vi "Actor Core.vi"(8 "error in":errorcluster, 11 "WS Test Client in":refnum<class "WS Test Client Subscriber.lvclass">) -> (0 "error out":errorcluster, 3 "Actor out":refnum<class "Actor.lvclass">)   [LabVIEW 2017, in "Echo Broadcast Test With Server Manager.lvlib" / "WS Test Client Subscriber.lvclass"]
doc: "(<B>Filename</B>: Actor Framework.lvlib:Actor.lvclass:Actor Core.vi)\n\nReceives messages to the actor, reacts to them, and initiates any error handling that may shut the actor down.\n\nDescendant classes may override this VI to append parallel tasks for the actor to complete while it handles messages. Overrides use the Call Parent Method node."
uses:
  WS Test Client Subscriber.lvclass
  C:/Program Files (x86)/National Instruments/LabVIEW 2017/vi.lib/ActorFramework/Actor/Actor.lvclass
  <vilib>/ActorFramework/Actor/Actor.lvclass
  <vilib>/ActorFramework/Message Enqueuer/Message Enqueuer.lvclass
  WebSocket Actor/WebSocket Client/WebSocket Client.lvclass
  C:/Projects/Shared Libraries/WebSocket Actor/WebSocket Actor/WebSocket Connection/WebSocket Connection.lvclass
  WS Test Client Subscriber Messages/Client Connection Handler Msg/Client Connection Handler Msg.lvclass
  C:/Projects/Shared Libraries/WebSocket Actor/WebSocket Actor/Abstract Messages/WebSocket Connection Handler Msg/WebSocket Connection Handler Msg.lvclass
  <vilib>/ActorFramework/Actor/Actor.lvclass/Actor.ctl
  <vilib>/ActorFramework/Message Enqueuer/Message Enqueuer.lvclass/Message Enqueuer.ctl
  WebSocket Actor/WebSocket Client/WebSocket Client.lvclass/WebSocket Client.ctl
  WebSocket Actor/WebSocket Connection/WebSocket Connection.lvclass/WebSocket Connection.ctl
  WS Test Client Subscriber.lvclass/WS Test Client Subscriber.ctl
  WebSocket Actor/WebSocket Client/properties/Write WS URI.vi
  WebSocket Actor/WebSocket Connection/properties/Write Timeout.vi
  WebSocket Actor/WebSocket Connection/properties/Write WebSocket Data Handler.vi
  <vilib>/ActorFramework/Message Enqueuer/Init from Existing Queue.vi
  <vilib>/ActorFramework/Message Enqueuer/Enqueue.vi
  <vilib>/ActorFramework/Stop Msg/Stop Msg.lvclass
  C:/Program Files (x86)/National Instruments/LabVIEW 2017/vi.lib/ActorFramework/Message/Message.lvclass
  <vilib>/ActorFramework/Message Priority Queue/Priority Enqueue.vi
  <vilib>/MGI/Monitored Actor/Monitored Actor/Monitored Actor/Monitored Actor.lvclass
  WebSocket Actor/WebSocket Connection Messages/Send to Peer Msg/Send to Peer Msg.lvclass
panel:
  in  "Send":bool
  in  "Data To Send":string
  in  "Exit":bool
  out "Echoed Data":string
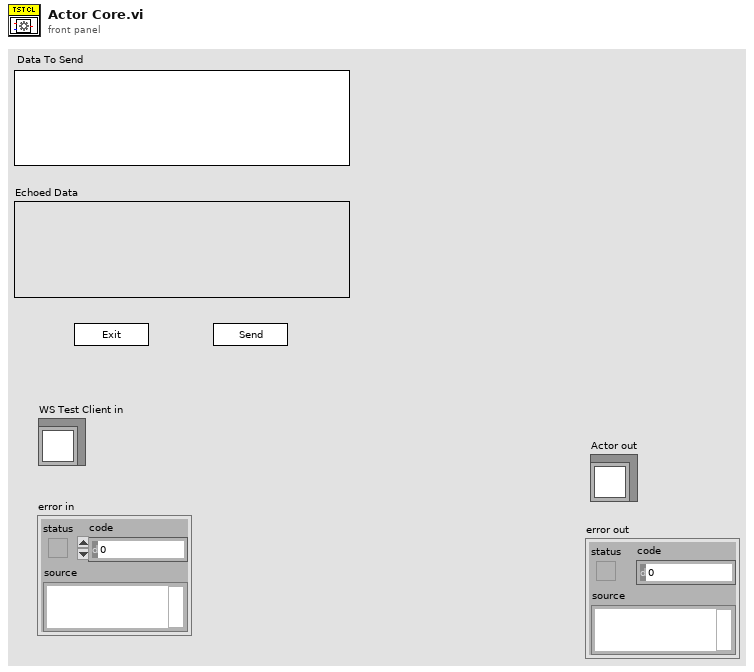
[diagram p1: front panel]
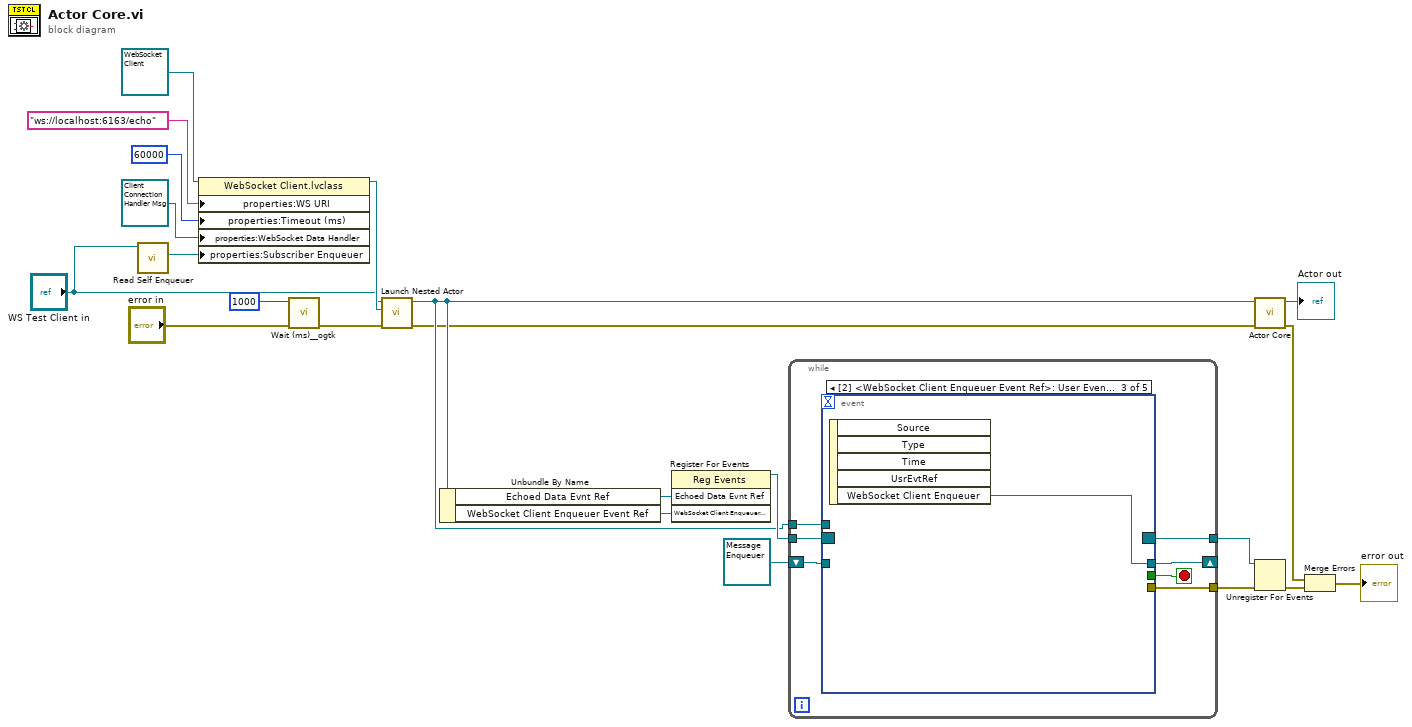
[diagram p0: block diagram]
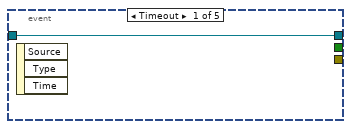
[diagram p2: hidden frame]
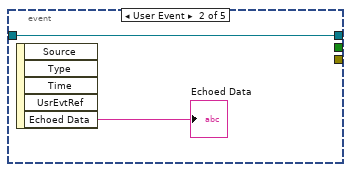
[diagram p3: hidden frame]
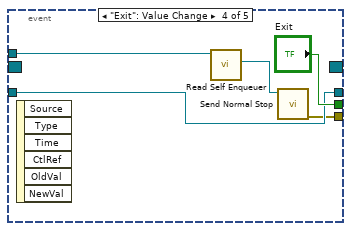
[diagram p4: hidden frame]
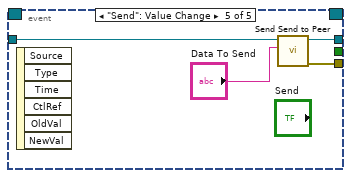
[diagram p5: hidden frame]
diagram:
  n1 = call <vilib>:"Read Self Enqueuer.vi"("Actor"="WS Test Client in") -> ("Self Enqueuer"=w5:refnum<class "Message Enqueuer.lvclass">)  [unwired: 10 in]
  n2 = property class="WebSocket Client.lvclass"(reference=refnum<class "WebSocket Client.lvclass"> refnum ("WebSocket Actors.lvlib:WebSocket Client.lvclass"), "properties:WS URI"="ws://localhost:6163/echo" ("Address"), "properties:Timeout (ms)"=60000 ("Timeout (60000 ms)"), "properties:WebSocket Data Handler"=refnum<class "Client Connection Handler Msg.lvclass"> refnum ("WS Full LabVIEW Test.lvlib:Client Connection Handler Msg.lvclass"), "properties:Subscriber Enqueuer"=w5) -> (reference out=w10:refnum<class "WebSocket Client.lvclass">)  [unwired: 1 in, 1 out]
  n3 = call <userlib>:"Wait (ms)__ogtk.vi"("error in (no error)"="error in", "milliseconds to wait"=u32 1000) -> ("error out"=w7:errorcluster)  [unwired: 8 in, 1 out]
  n4 = call <vilib>:"Launch Nested Actor.vi"("error in (no error)"=w7, "Nested Actor"=w10, "Caller Actor in"="WS Test Client in") -> ("error out"=w1:errorcluster, "Caller Actor out"=w2:refnum<class "WS Test Client Subscriber.lvclass">)  [unwired: 6 in, 1 out]
  n5 = Unbundle By Name(w2) -> ("Echoed Data Evnt Ref"=w20:refnum<user-event>, "WebSocket Client Enqueuer Event Ref"=w18:refnum<user-event>)
  n6 = register-events(w20, w18) -> (reference out=w19:refnum<event-registration>)  [unwired: 2 in, 1 out]
  n7 = while {
    tunnel: w19 -> [w29]
    shift-right: [w27] -> _
    shift-left: refnum<class "Message Enqueuer.lvclass"> refnum ("WebSocket Client Enqueuer") -> [w26]
    tunnel: [w25] -> w16
    tunnel: w2 -> [w24]
    tunnel: [w23] -> w13
    stop <- w28 stop-if-true
    n8 = event shown="[2] <WebSocket Client Enqueuer Event Ref>: User Event" {
      selector: w29 -> [_ _ _ _ _]
      dyn-events: [_ _ _ _ _] -> w25
      timeout: _ -> [_ _ _ _ _]
      tunnel: [_ _ _ "Exit" _] -> w28
      tunnel: [w30 w31 w33 w37 w40] -> w27
      tunnel: w26 -> [w30 w31 _ w37 w41]
      tunnel: w24 -> [_ _ _ w36 _]
      tunnel: [_ _ _ w34 w39] -> w23
      event Timeout {
        n9 = event-data() -> ()  [unwired: 1 in, 3 out]
      }
      event User Event {
        n10 = event-data() -> ("Echoed Data"=→"Echoed Data":string)  [unwired: 1 in, 4 out]
      }
      event User Event {
        n11 = event-data() -> ("WebSocket Client Enqueuer"=w33:refnum<class "Message Enqueuer.lvclass">)  [unwired: 1 in, 4 out]
      }
      event "Exit": Value Change {
        n12 = event-data() -> ()  [unwired: 1 in, 6 out]
        n13 = call <vilib>:"Read Self Enqueuer.vi"("Actor"=w36) -> ("Self Enqueuer"=w35:refnum<class "Message Enqueuer.lvclass">)  [unwired: 10 in]
        n14 = call <vilib>:"Send Normal Stop.vi"("Message Enqueuer"=w35) -> ("error out"=w34:errorcluster)  [unwired: 10 in]
      }
      event "Send": Value Change {
        n15 = event-data() -> ()  [unwired: 1 in, 6 out]
        n16 = call "Send Send to Peer.vi"("Data"="Data To Send", "Message Enqueuer in"=w41) -> ("error out"=w39:errorcluster, "Message Enqueuer out"=w40:refnum<class "Message Enqueuer.lvclass">)  [unwired: 8 in]
      }
    }
  }
  n17 = call-parent "Actor Core.vi"("error in"=w1, "Actor in"=w2) -> ("error out"=w22:errorcluster, "Actor out"=→"Actor out":refnum<class "Actor.lvclass">)  [unwired: 8 in]
  n18 = Unregister For Events(event registration refnum=w16, error in=w13) -> (error out=w14:errorcluster)
  n19 = Merge Errors(w22, w14) -> (→"error out":errorcluster)
